vi "Read SSL Protocols.vi"(8 "error in (no error)":errorcluster, 11 "dotNET SSL Socket in":refnum<class "dotNET SSL Socket.lvclass">) -> (0 "error out":errorcluster, 2 "SSL Protocols":i32[](array[ring])=[240] items=["None"=0, "Ssl2"=12, "Ssl3"=48, "Tls"=192, "Default"=240, "Tls11"=768, "Tls12"=3072], 3 "dotNET SSL Socket out":refnum<class "dotNET SSL Socket.lvclass">)   [LabVIEW 2013, in "dotNET SSL Socket.lvlib" / "dotNET SSL Socket.lvclass"]
uses:
  dotNET SSL Socket.lvclass
  dotNET SSL Socket.lvclass/dotNET SSL Socket.ctl
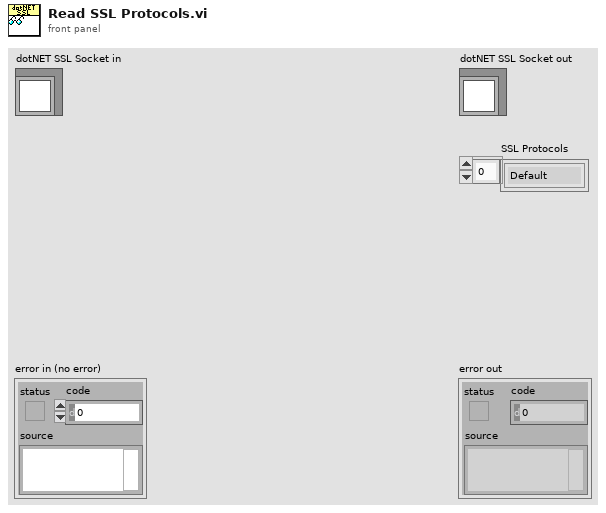
[diagram p1: front panel]
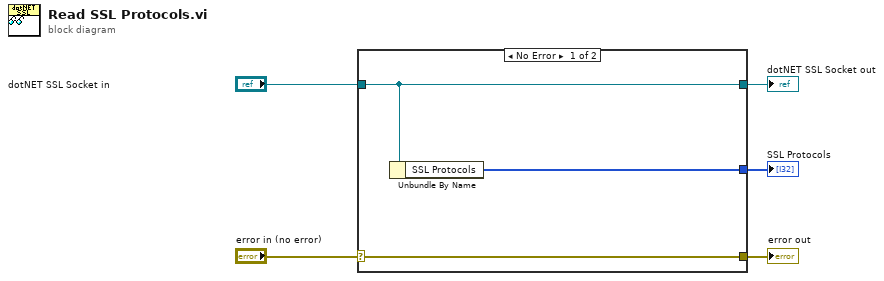
[diagram p0: block diagram]
diagram:
  n1 = case shown="No Error" "error in (no error)" {
    selector: "error in (no error)" -> [w8 w9]
    tunnel: [w8 w9] -> w4
    tunnel: [w7 w10] -> w2
    tunnel: "dotNET SSL Socket in" -> [w7 w10]
    tunnel: [w6 _] -> w1
    frame No Error {
      n2 = Unbundle By Name(w7) -> ("SSL Protocols"=w6:i32[])
    }
    frame Error {
    }
  }
  "error out" <- w4
  "dotNET SSL Socket out" <- w2
  "SSL Protocols" <- w1
